vi "_utils_ Remove EOI Warning.vi"(0 "error in":errorcluster) -> (1 "Ending character read?":bool, 2 "error out":errorcluster)   [LabVIEW 2014]
doc: "If 1073676293 VISA warning was returned (the specified termination character was read) replaces it with \"No Error\"."
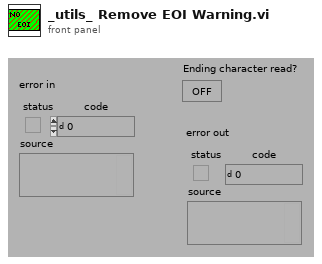
[diagram p1: front panel]
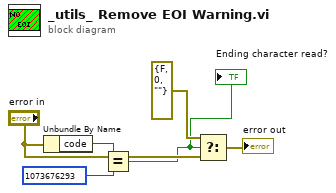
[diagram p0: block diagram]
diagram:
  n1 = Unbundle By Name("error in") -> ("code"=w2:i32)
  n2 = Equal?(x=w2, y=1073676293) -> (x = y?=w1:bool)
  "Ending character read?" <- w1
  n3 = Select(t=errorcluster {"status"=FALSE, "code"=0, "source"=""}, s=w1, f="error in") -> (s? t:f=→"error out":errorcluster)
